vi "FIR_2Decimate_FilterBank.vi"(8 "data valid in":bool, 9 "Q in":fxp<+/-,16,14>[](array[numeric])=[0.0, 0.0], 10 "I in":fxp<+/-,16,14>[](array[numeric])=[0.0, 0.0]) -> (0 "data valid out":bool, 1 "Q out":fxp<+/-,16,14>, 2 "I out":fxp<+/-,16,14>)   [LabVIEW 2013]
uses:
  <vilib>/rvi/FXPMathLib/FxpConvert/subVIs/nifxpmath_Convert_SimConfig.ctl
  <vilib>/fxp/LVFixedPointQuantizationPolicyTypeDef.ctl
  <vilib>/fxp/LVFixedPointOverflowPolicyTypeDef.ctl
  <vilib>/rvi/FXPMathLib/FxpConvert/simVIs/DllFxpConvertTemp_sub.vi
  <vilib>/rvi/FXPMathLib/FxpInterpret/XNode/nifxpmath_Interpret.xnode
  <vilib>/rvi/FXPMathLib/FxpConvert/XNode/nifxpmath_Convert.xnode
  <vilib>/rvi/FXPMathLib/FxpAdd/XNode/nifxpmath_Add.xnode
  <vilib>/rvi/FXPMathLib/sim/FxpSim.dll
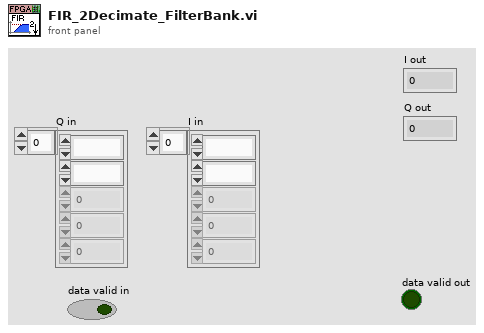
[diagram p1: front panel]
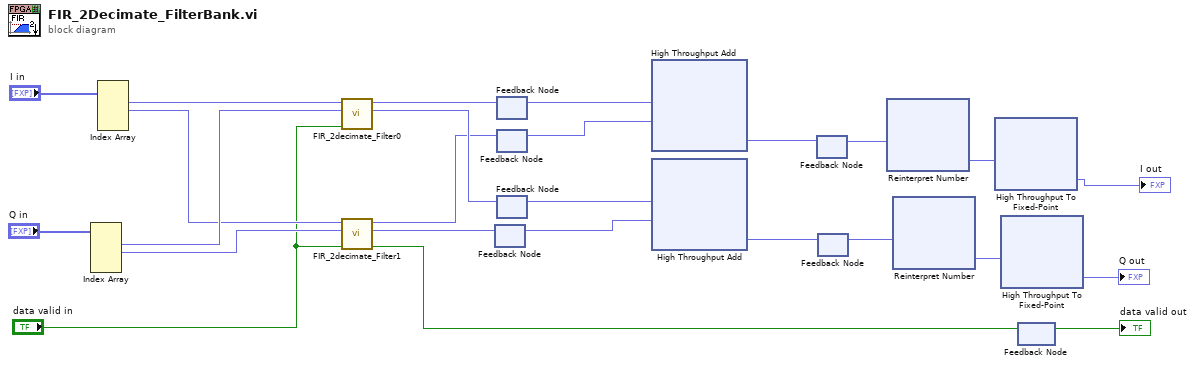
[diagram p0: block diagram]
diagram:
  n1 = Index Array(array="Q in") -> (element #1=w18:fxp<+/-,16,14>, element #2=w16:fxp<+/-,16,14>)  [unwired: 4 in, 2 out]
  n2 = Index Array(array="I in") -> (element #1=w21:fxp<+/-,16,14>, element #2=w17:fxp<+/-,16,14>)  [unwired: 4 in, 2 out]
  n3 = call "FIR_2decimate_Filter0.vi"("valid in"="data valid in", "Q in"=w18, "I in"=w21) -> ("Q out"=w14:fxp<+/-,16,14>, "I out"=w2:fxp<+/-,16,14>)  [unwired: 6 in, 1 out]
  n4 = call "FIR_2decimate_Filter1.vi"("valid in"="data valid in", "Q in"=w16, "I in"=w17) -> ("valid out"=w5:bool, "Q out"=w12:fxp<+/-,16,14>, "I out"=w13:fxp<+/-,16,14>)  [unwired: 6 in]
  n5 = feedback #1() -> (w22:fxp<+/-,16,14>)  [unwired: 1 in]
  n6 = feedback-in #1(w12) -> ()
  n7 = feedback #2() -> (w25:fxp<+/-,16,14>)  [unwired: 1 in]
  n8 = feedback-in #2(w2) -> ()
  n9 = feedback #3() -> (w24:fxp<+/-,16,14>)  [unwired: 1 in]
  n10 = feedback-in #3(w13) -> ()
  n11 = feedback #4() -> (w23:fxp<+/-,16,14>)  [unwired: 1 in]
  n12 = feedback-in #4(w14) -> ()
  n13 = xnode ("High Throughput Add")("x"=w25, "y"=w24) -> ("x+y"=w4:fxp<+/-,19,15>)
  n14 = xnode ("High Throughput Add")("x"=w23, "y"=w22) -> ("x+y"=w3:fxp<+/-,19,15>)
  n15 = feedback #5() -> (w9:fxp<+/-,19,15>)  [unwired: 1 in]
  n16 = feedback-in #5(w4) -> ()
  n17 = feedback #6() -> (w7:fxp<+/-,19,15>)  [unwired: 1 in]
  n18 = feedback-in #6(w3) -> ()
  n19 = xnode "Reinterpret Number"("x"=w9) -> ("y"=w10:fxp<+/-,19,14>)
  n20 = xnode "Reinterpret Number"("x"=w7) -> ("y"=w8:fxp<+/-,19,14>)
  n21 = xnode ("High Throughput To Fixed-Point")("x"=w10) -> ("y"=→"I out":fxp<+/-,16,14>)
  n22 = xnode ("High Throughput To Fixed-Point")("x"=w8) -> ("y"=→"Q out":fxp<+/-,16,14>)
  n23 = feedback #7() -> (→"data valid out":bool)  [unwired: 1 in]
  n24 = feedback-in #7(w5) -> ()
